vi "Poly_InitTimer.vi"   [LabVIEW 2012]
doc: "Initializes the timer associated with the unique \"Timer\" value."
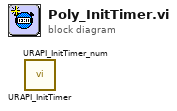
[diagram p0: block diagram]
diagram:
  n1 = call <userlib>:"URAPI_InitTimer.vi"() -> ()  [unwired: 4 in, 2 out]
  n2 = call <userlib>:"URAPI_InitTimer_num.vi"() -> ()  [unwired: 4 in, 2 out]
